vi "Lock.vi"(0 "Interface_object in":refnum<class "Timed Door.lvclass">, 5 "error in (no error)":errorcluster) -> (14 "Interface_object out":refnum<class "Timed Door.lvclass">, 19 "error out":errorcluster)   [LabVIEW 2018, in "Timed Door.lvclass"]
uses:
  Timed Door.lvclass
  Timed Door.lvclass/Timed Door.ctl
  Get Door.vi
  Set Door.vi
  Get Alarm DVR.vi
  Door/Door.lvclass
  Alarm/Alarm.lvclass
  Timer/Timer.lvclass
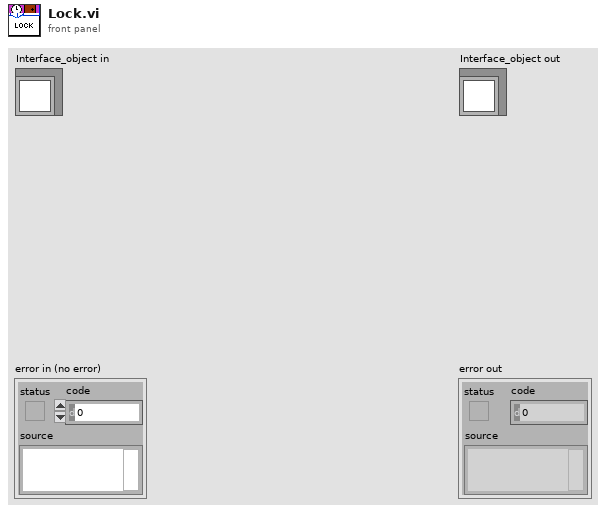
[diagram p1: front panel]
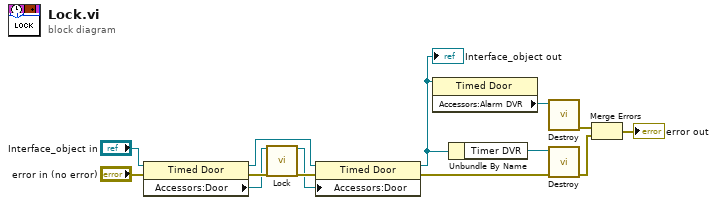
[diagram p0: block diagram]
diagram:
  n1 = property class="Timed Door"(reference="Interface_object in", error in="error in (no error)") -> (reference out=w8:refnum<class "Timed Door.lvclass">, error out=w14:errorcluster, "Accessors:Door"=w10:refnum<class "Door.lvclass">)
  n2 = call-dynamic "Lock.vi"("Interface_object in"=w10, "error in (no error)"=w14) -> ("Interface_object out"=w9:refnum<class "Door.lvclass">, "error out"=w13:errorcluster)  [unwired: 16 in]
  n3 = property class="Timed Door"(reference=w8, error in=w13, "Accessors:Door"=w9) -> (reference out=w3:refnum<class "Timed Door.lvclass">, error out=w2:errorcluster)
  "Interface_object out" <- w3
  n4 = property class="Timed Door"(reference=w3) -> ("Accessors:Alarm DVR"=w5:refnum<data-value>)  [unwired: 1 in, 2 out]
  n5 = Unbundle By Name(w3) -> ("Timer DVR"=w6:refnum<data-value>)
  n6 = call "Destroy.vi"("Alarm DVR"=w5) -> ("error out"=w4:errorcluster)  [unwired: 10 in]
  n7 = call "Destroy.vi"("error in (no error)"=w2, "Timer DVR"=w6) -> ("error out"=w7:errorcluster)  [unwired: 9 in]
  n8 = Merge Errors(w4, w7) -> (→"error out":errorcluster)
